vi "Calculate Color Index Array.vi"(8 "error in (no error)":errorcluster, 10 "3D Scatter Datatype in":refnum<class "3D Scatter Datatype.lvclass">, 11 "Plot Representation In":T1) -> (0 "error out":errorcluster, 2 "3D Scatter Datatype out":refnum<class "3D Scatter Datatype.lvclass">, 3 "Plot Representation Out":T1)   [LabVIEW 2020, in "3D Scatter Datatype.lvclass"]
uses:
  <vilib>/Math Plots/3D Math Plots/3D Scatter/3D Scatter Datatype/3D Scatter Datatype.lvclass
  <vilib>/Math Plots/3D Math Plots/3D Plot/3D Plot/Typedef/Plot Representation.ctl
  <vilib>/Math Plots/3D Math Plots/3D Plot/3D Plot/Typedef/Range Clusters.ctl
  <vilib>/Math Plots/3D Math Plots/3D Plot/3D Plot/Typedef/Mesh Data.ctl
  <vilib>/Math Plots/3D Math Plots/3D Scatter/3D Scatter Datatype/3D Scatter Datatype.lvclass/3D Scatter Datatype.ctl
  <vilib>/Math Plots/3D Math Plots/3D Plot/3D Plot Datatype/3D Plot Datatype.lvclass
  <vilib>/Math Plots/3D Math Plots/3D Plot/3D Plot/3D Plot.lvclass
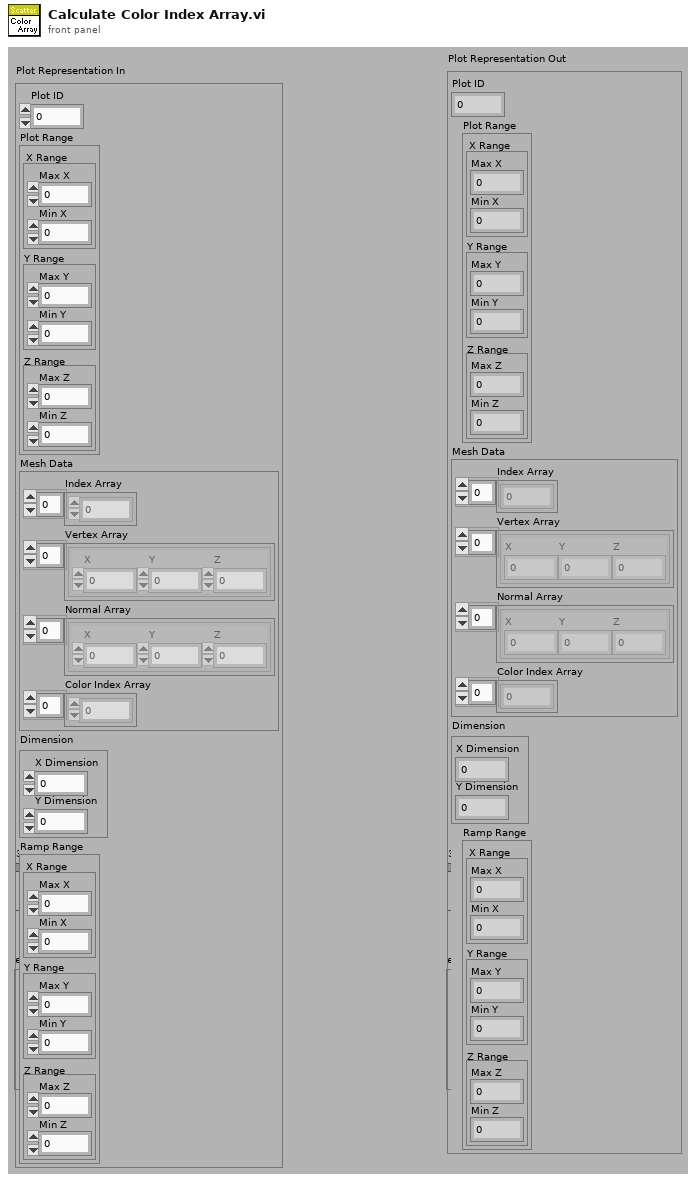
[diagram p1: front panel]
types:
  T1 = typedef "3D Plot.lvclass/Plot Representation.ctl" = cluster{"Plot ID":i32, "Plot Range":T2, "Mesh Data":T3, "Dimension":cluster{"X Dimension":i32, "Y Dimension":i32}, "Ramp Range":T2}
  T2 = typedef "3D Plot.lvclass/Range Clusters.ctl" = cluster{"X Range":cluster{"Max X":sgl, "Min X":sgl}, "Y Range":cluster{"Max Y":sgl, "Min Y":sgl}, "Z Range":cluster{"Max Z":sgl, "Min Z":sgl}}
  T3 = typedef "3D Plot.lvclass/Mesh Data.ctl" = cluster{"Index Array":u32[], "Vertex Array":cluster{"X":sgl, "Y":sgl, "Z":sgl}[], "Normal Array":cluster{"X":sgl, "Y":sgl, "Z":sgl}[], "Color Index Array":i32[]}
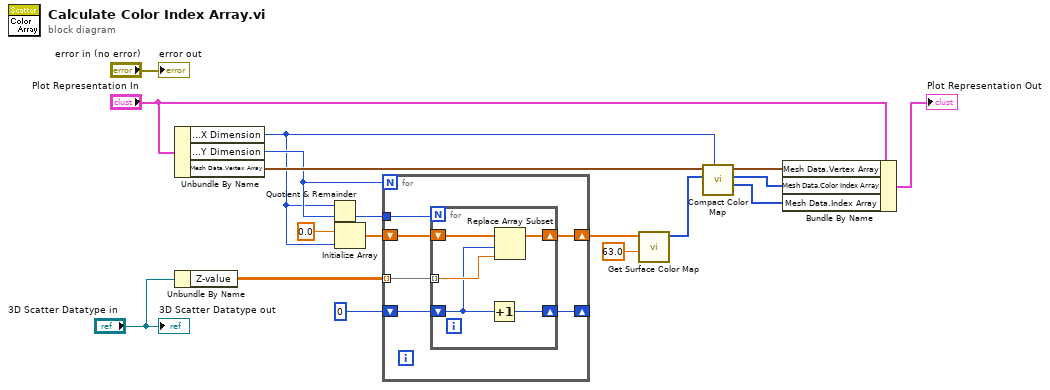
[diagram p0: block diagram]
diagram:
  n1 = Unbundle By Name("Plot Representation In") -> ("Dimension.X Dimension"=w1:i32, "Dimension.Y Dimension"=w3:i32, "Mesh Data.Vertex Array"=w12:cluster{"X":sgl, "Y":sgl, "Z":sgl}[])
  n2 = Unbundle By Name("3D Scatter Datatype in") -> ("Z-value"=w8:sgl[][])
  n3 = Quotient & Remainder(x=w1, y=w3) -> (floor(x/y)=w2:i32)  [unwired: 1 out]
  n4 = Initialize Array(sgl 0.0 ("element"), w1) -> (w10:sgl[])
  n5 = for {
    N: w3 -> [_]
    shift-right: [w20] -> w7
    shift-left: w10 -> [w24]
    tunnel: w8 -> [w23] mode=indexing
    shift-right: [w22] -> _
    shift-left: 0 -> [w21]
    tunnel: w2 -> [w19]
    n6 = for {
      N: w19 -> [_]
      shift-right: [w28] -> w20
      shift-left: w24 -> [w29]
      tunnel: w23 -> [w27] mode=indexing
      shift-right: [w26] -> w22
      shift-left: w21 -> [w25]
      n7 = Increment(x=w25) -> (x+1=w26:i32)
      n8 = Replace Array Subset(array=w29, new element=w27, index=w25) -> (w28:sgl[])
    }
  }
  n9 = call <vilib>:"Get Surface Color Map.vi"("Levels"=sgl 63.0, "Amplifiy"=w7) -> ("Color Index Array"=w16:i32[])  [unwired: 9 out]
  n10 = call <vilib>:"Compact Color Map.vi"("X Dimension"=w1, "Color Index Array In"=w16, "Vertex Array In"=w12) -> ("Index for Same Color Vertex"=w13:u32[], "Compact Color Index Array Out"=w14:i32[], "Reordered Vertex Array Out"=w15:cluster{"X":sgl, "Y":sgl, "Z":sgl}[])  [unwired: 3 in, 3 out]
  n11 = Bundle By Name(cluster="Plot Representation In", "Mesh Data.Vertex Array"=w15, "Mesh Data.Color Index Array"=w14, "Mesh Data.Index Array"=w13) -> (→"Plot Representation Out":T1)
  "error out" <- "error in (no error)"
  "3D Scatter Datatype out" <- "3D Scatter Datatype in"
